vi "7-Segment_Simulator.vi"() -> ()   [LabVIEW 2024]
panel:
  in  "Stop":bool
  in  "Input":u8
  out "7 Seg.Display":T1
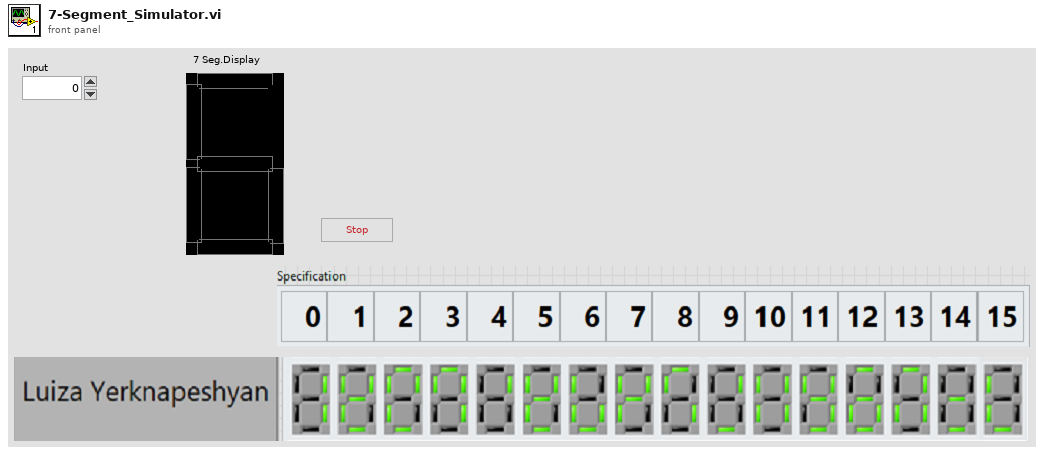
[diagram p1: front panel]
types:
  T1 = cluster{"a":bool, "b":bool, "c":bool, "d":bool, "e":bool, "f":bool, "g":bool}
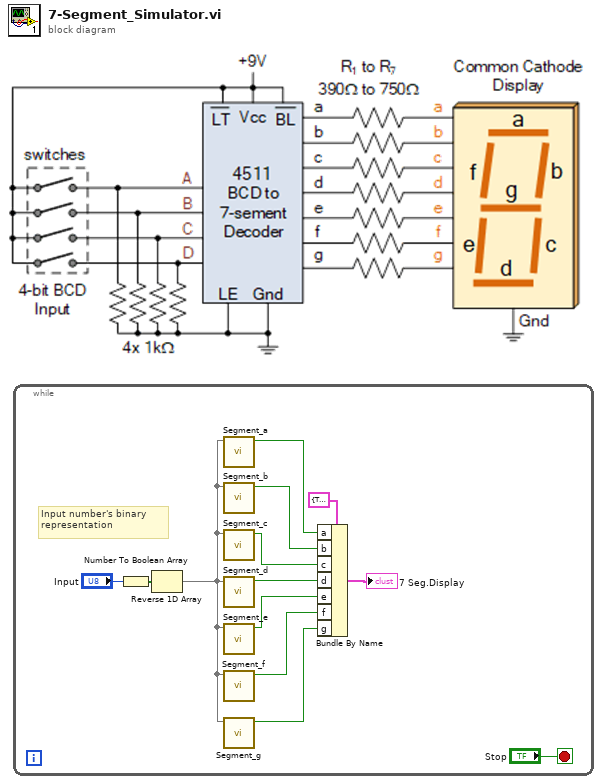
[diagram p0: block diagram]
diagram:
  n1 = while {
    stop <- "Stop" stop-if-true
    # "Input number's binary representation"
    n2 = Number To Boolean Array(number="Input") -> (Boolean array=w12:bool[])
    n3 = Reverse 1D Array(array=w12) -> (reversed array=w1:bool[])
    n4 = call "Segment_a.vi"("Input in Binary"=w1) -> ("Segment a"=w8:bool)  [unwired: 10 in]
    n5 = call "Segment_b.vi"("Input in Binary"=w1) -> ("Segment b"=w7:bool)  [unwired: 10 in]
    n6 = call "Segment_c.vi"("Input in Binary"=w1) -> ("Segment c"=w6:bool)  [unwired: 10 in]
    n7 = call "Segment_d.vi"("Input in Binary"=w1) -> ("Segment d"=w5:bool)  [unwired: 10 in]
    n8 = call "Segment_e.vi"("Input in Binary"=w1) -> ("Segment e"=w4:bool)  [unwired: 10 in]
    n9 = call "Segment_f.vi"("Input Iin Binary"=w1) -> ("Segment f"=w3:bool)  [unwired: 10 in]
    n10 = call "Segment_g.vi"("Boolean Array"=w1) -> ("Segment g"=w2:bool)  [unwired: 10 in]
    n11 = Bundle By Name(cluster=T1 {"a"=TRUE, "b"=TRUE, "c"=TRUE, "d"=TRUE, "e"=TRUE, "f"=TRUE, "g"=TRUE} ("Display"), "a"=w8, "b"=w7, "c"=w6, "d"=w5, "e"=w4, "f"=w3, "g"=w2) -> (→"7 Seg.Display":T1)
  }
